vi "waardes neighbours.vi"(10 "ArrayNeighbours":i32[][](array[numeric]), 11 "Array Dead Or Allive":u32[][](array[numeric])) -> (3 "Array":u32[](array[numeric]))   [LabVIEW 2013]
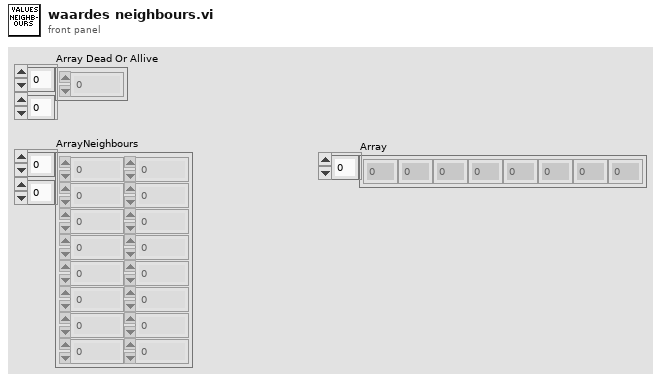
[diagram p1: front panel]
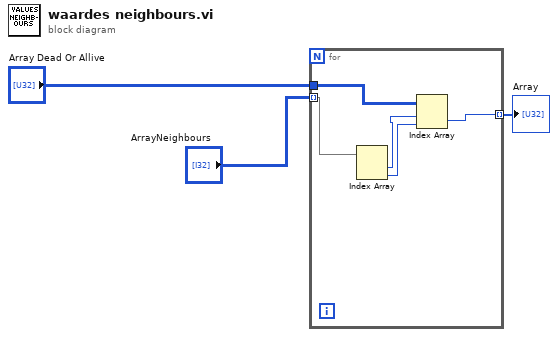
[diagram p0: block diagram]
diagram:
  n1 = for {
    tunnel: "ArrayNeighbours" -> [w7] mode=indexing
    tunnel: "Array Dead Or Allive" -> [w8]
    tunnel: [w6] -> w1 mode=indexing
    n2 = Index Array(array=w7) -> (element #1=w4:i32, element #2=w5:i32)  [unwired: 2 in]
    n3 = Index Array(array=w8, index (row)=w4, index (col)=w5) -> (element=w6:u32)
  }
  "Array" <- w1
